vi "encoder_debug_v1.vi"() -> ()   [LabVIEW 2014]
uses:
  <vilib>/LabVIEW Targets/FPGA/cRIO/shared/nicrio_ModuleControls/nicrio_cRIO-9237_DataRatesRing.ctl
  <vilib>/LabVIEW Targets/FPGA/cRIO/shared/nicrio_ModuleControls/nicrio_cRIO-9237_ExcitationVoltageRing.ctl
  <vilib>/rvi/FXPMathLib/FxpSinAndCos/subVIs/nifxpmath_SinAndCos_SimConfig.ctl
  <vilib>/rvi/Emulation/niFpgaGetClockAttributes.vi
  <vilib>/rvi/Emulation/niFpgaSctlEmulationGetInTimedLoop.vi
  <vilib>/rvi/Emulation/niFpgaEmulationReportErrorSimple.vi
  <vilib>/rvi/Emulation/niFpgaProcessEmulError.vi
  <vilib>/rvi/interface/RandomDataEmulation/nirviRandomDataMultiElementFPGAFIFO.vi
  <instcachedir>/0/nirviRandomDataMultiElementFPGAFIFO_AD0CFC12EF974623A9C2E4184BC062B2.lvgen/nirviRandomDataMultiElementFPGAFIFO_AD0CFC12EF974623A9C2E4184BC062B2_025.vi
  <vilib>/rvi/interface/RandomDataEmulation/niFpgaRandomDataHandleErrors.vi
  <vilib>/rvi/Emulation/niFpgaCriticalErrorInLSC.vi
  <vilib>/rvi/FXPMathLib/FxpSinAndCos/simVIs/DllFxpSinAndCosTemp_sub.vi
  <vilib>/rvi/eio/common/nirviEmuTemplateMethod_errors.vi
  <vilib>/rvi/eio/common/nirviEmuTemplatePropertySet_errors.vi
  <vilib>/rvi/DataTransferAndStorage/Container/XNode/niFpgaContainer.xnode
  <vilib>/rvi/interface/RandomDataEmulation/nirviRandomDataFpgaMultiElementTemplate.vi
  <vilib>/rvi/FXPMathLib/FxpSinAndCos/XNode/nifxpmath_SinAndCos.xnode
  <vilib>/rvi/Analysis/measure/butterworth/XNode/niFpgaButterworthFilter.xnode
  <vilib>/eio/EIONode/EIONode.xnode
  <vilib>/eio/EIOPropertyNode/EIOPropertyNode.xnode
  <vilib>/rvi/eio/common/nirviEmuTemplatePropertyGet_errors.vi
  <vilib>/rvi/eio/common/nirviEmuTemplatePropertyGet_noerrors.vi
  <vilib>/rvi/eio/common/nirviEmuTemplatePropertySet_noerrors.vi
panel:
  out "omega_p2 (rad/s)":fxp<+/-,36,13>
  out "Dp2_d (mm/s)":fxp<+/-,36,13>
  out "omega_p2 (Mavg)":fxp<+/-,36,14>
  out "Dp2_d (Mavg)":fxp<+/-,36,14>
  in  "mt0_p2":u32
  out "Dp2_d (Mavg w. f.)":fxp<+/-,36,14>
  out "Dp1_d (Mavg w. f.)":fxp<+/-,36,14>
  in  "Dp_d (Mavg) coeff.":i32[](array[numeric])=[946630756, 63555534]
  in  "Dy_d (Mavg) coeff.":i32[](array[numeric])=[946630756, 63555534]
  out "omega_p2 (Mavg w. f.)":fxp<+/-,36,14>
  in  "omega_y(Mavg) coeff.":i32[](array[numeric])=[946630756, 63555534]
  out "omega_p1 (Mavg w. f)":fxp<+/-,36,14>
  in  "omega_P(Mavg) coeff.":i32[](array[numeric])=[946630756, 63555534]
  in  "FIFO":i16(ring) items=["Pitch_F+P", "imp ctrl", "Yaw_F+P"]
  out "PID (kHz)":fxp<+/-,20,10>
  in  "Set 6":bool
  in  "Set 5":bool
  in  "Set 4":bool
  in  "Set 3":bool
  in  "Set 2":bool
  in  "Set 1":bool
  out "Dp1_d (T)":fxp<+/-,36,13>
  out "omega_p1 (T)":fxp<+/-,36,13>
  out "Dp2_d (T)":fxp<+/-,36,13>
  out "omega_p2 (T)":fxp<+/-,36,13>
  out "mt_omega_p2":u32
  out "Encoder Position_p2":i32
  out "D_p2":fxp<+/-,32,7>
  out "rad_p2":fxp<+/-,33,20>
  out "D_p1":fxp<+/-,32,7>
  out "rad_p1":fxp<+/-,33,20>
  out "Encoder Position_p1":i32
  out "Dp1_d (Mavg)":fxp<+/-,36,14>
  out "omega_p1 (Mavg)":fxp<+/-,36,14>
  in  "Dp_d_M_avg_Tc (uSec)":i32
  in  "Vp. Est.":i16(ring) items=["T", "Mavg", "Mavg w. f."]
  in  "Mag. factor_p":fxp<+/-,20,3>
  in  "Belt_out_p":fxp<+/-,7,7>
  in  "Belt_in_p":fxp<+/-,6,6>
  out "Fp_dc":fxp<+/-,32,10>
  in  "Zero_p":bool
  in  "mt0_p1":u32
  in  "Dp_dd coeff.":i32[](array[numeric])=[946630756, 63555534]
  out "Dp_dd":fxp<+/-,36,25>
  out "dFp_PID":fxp<+/-,36,18>
  in  "dFp_PID coeff.":i32[](array[numeric])=[946630756, 63555534]
  out "fpt_i":fxp<+/-,34,18>
  out "Dpr_sin":fxp<+/-,22,7>
  in  "Sin offset_p":fxp<+/-,22,7>
  in  "Sin magnitude_p":fxp<+/-,21,6>
  out "Dpr_sin_dd":fxp<+/-,35,20>
  out "Dpr_sin_d":fxp<+/-,33,15>
  out "Sin omega_p":fxp<+/-,34,9>
  in  "Sin wave freq._p (Hz)":fxp<+/-,32,6>
  in  "Dpr_step":fxp<+/-,22,7>
  out "Dpr_for":fxp<+/-,22,7>
  in  "Command_p":i16(ring) items=["Step", "Sine"]
  in  "Ki_p":fxp<+/-,30,9>
  out "Fp_PID":fxp<+/-,36,16>
  in  "fp_tolorance":fxp<+,22,6>
  out "fp_tilde":fxp<+/-,33,10>
  in  "Kp_p":fxp<+/-,32,13>
  out "Fr_p":fxp<+/-,32,10>
  in  "S/F coeff_p":fxp<+/-,25,-10>
  out "va_p1":fxp<+/-,36,7>
  out "vb_p1":fxp<+/-,37,8>
  out "vq_p2_F":fxp<+/-,20,5> format="%.57g"
  out "vd_p2_F":fxp<+/-,20,5>
  in  "Stop motor_p":bool
  out "Force_p":fxp<+/-,32,10>
  in  "Strain selection_p":i16(ring) items=["Raw", "Avg.8", "Avg.8 w. filter"]
  out "Strain_p (Avg8 w. f)":fxp<+/-,36,8>
  in  "Strain_p Avg.8 coeff.":i32[](array[numeric])=[946630756, 63555534]
  out "Strain_p (Avg8)":fxp<+/-,36,4>
  out "Raw Strain_p":fxp<+/-,36,4>
  out "Mod6/AI3":fxp<+/-,36,4>
  in  "Strain gage reset_p":bool
  out "Dp1_d (mm/s)":fxp<+/-,36,13>
  out "omega_p1 (rad/s)":fxp<+/-,36,13>
  out "mt_omega_p1":u32
  in  "Encoder reset_p":bool
  out "Strain_y (Avg8 w. f)":fxp<+/-,36,8>
  in  "Strain_y Avg8 coeff.":i32[](array[numeric])=[-898916953, 1957103773, 3888751]
  out "Strain_y (Avg8)":fxp<+/-,36,4>
  out "vb_p2":fxp<+/-,38,8>
  out "va_p2":fxp<+/-,38,8>
  out "Time now(s)":fxp<+,52,14>
  out "vq_p1_F":fxp<+/-,20,5> format="%.57g"
  out "vd_p1_F":fxp<+/-,20,5>
  in  "Stop motor_y":bool
  in  "Ini coe.":bool
  out "Loop rate (kHz)":fxp<+/-,36,7>
  out "Raw Strain_y":fxp<+/-,36,4>
  in  "Strain gage reset_y":bool
  in  "Stop (Strain)":bool
  out "Mod6/AI2":fxp<+/-,36,4>
  in  "Excitation Voltage":T1 items=["2.5 Volts", "3.3 Volts", "5.0 Volts", "10.0 Volts", "External Excitation"]
  in  "Data Rate":T2=1 items=["50.000 kS/s (NI 9237)"=1, "25.000 kS/s (NI 9237)"=2, "16.667 kS/s (NI 9237)"=3, "12.500 kS/s (NI 9237)"=4, "10.000 kS/s (NI 9237)"=5, "8.333 kS/s (NI 9237)"=6, "7.143 kS/s (NI 9237)"=7, "6.250 kS/s (NI 9237)"=8, "5.556 kS/s (NI 9237)"=9, "5.000 kS/s (NI 9237)"=10, "4.545 kS/s (NI 9237)"=11, "4.167 kS/s (NI 9237)"=12, "3.846 kS/s (NI 9237)"=13, "3.571 kS/s (NI 9237)"=14, "3.333 kS/s (NI 9237)"=15, "3.125 kS/s (NI 9237)"=16, "2.941 kS/s (NI 9237)"=17, "2.778 kS/s (NI 9237)"=18, "2.632 kS/s (NI 9237)"=19, "2.500 kS/s (NI 9237)"=20, "2.381 kS/s (NI 9237)"=21, "2.273 kS/s (NI 9237)"=22, "2.174 kS/s (NI 9237)"=23, "2.083 kS/s (NI 9237)"=24, "2.000 kS/s (NI 9237)"=25, "1.923 kS/s (NI 9237)"=26, "1.852 kS/s (NI 9237)"=27, "1.786 kS/s (NI 9237)"=28, "1.724 kS/s (NI 9237)"=29, "1.667 kS/s (NI 9237)"=30, "1.613 kS/s (NI 9237)"=31]
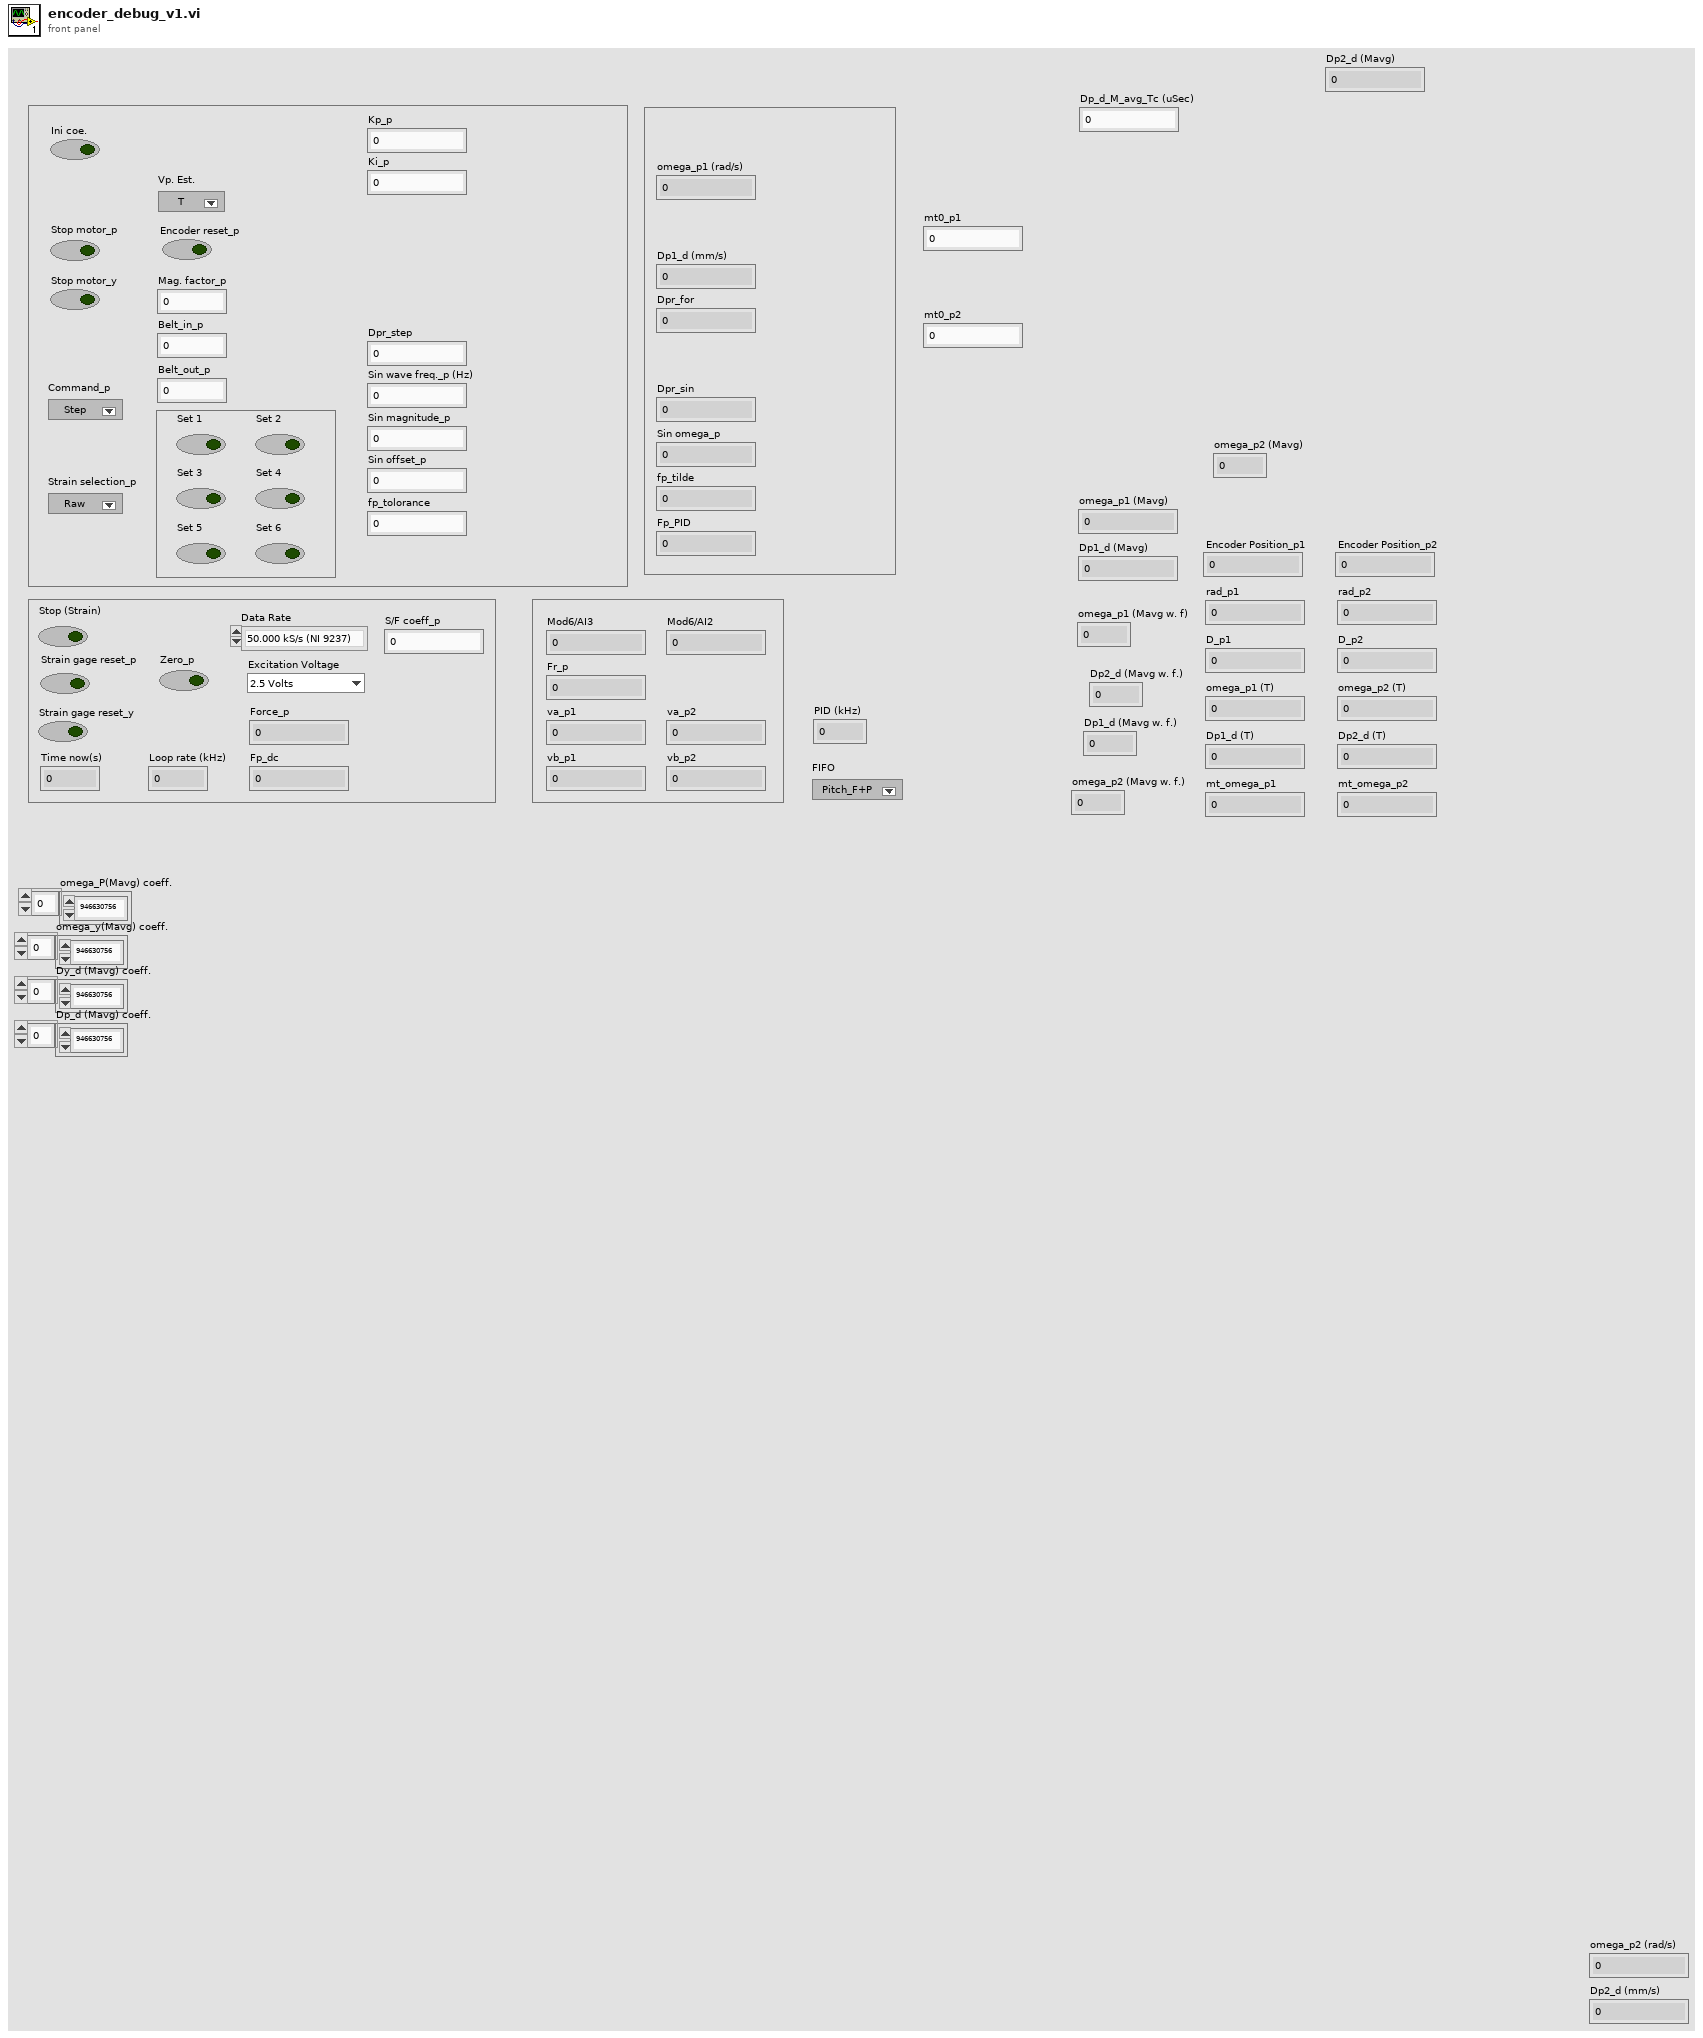
[diagram p1: front panel]
types:
  T1 = typedef "nicrio_cRIO-9237_ExcitationVoltageRing.ctl" = u8
  T2 = typedef "nicrio_cRIO-9237_DataRatesRing.ctl" = u8
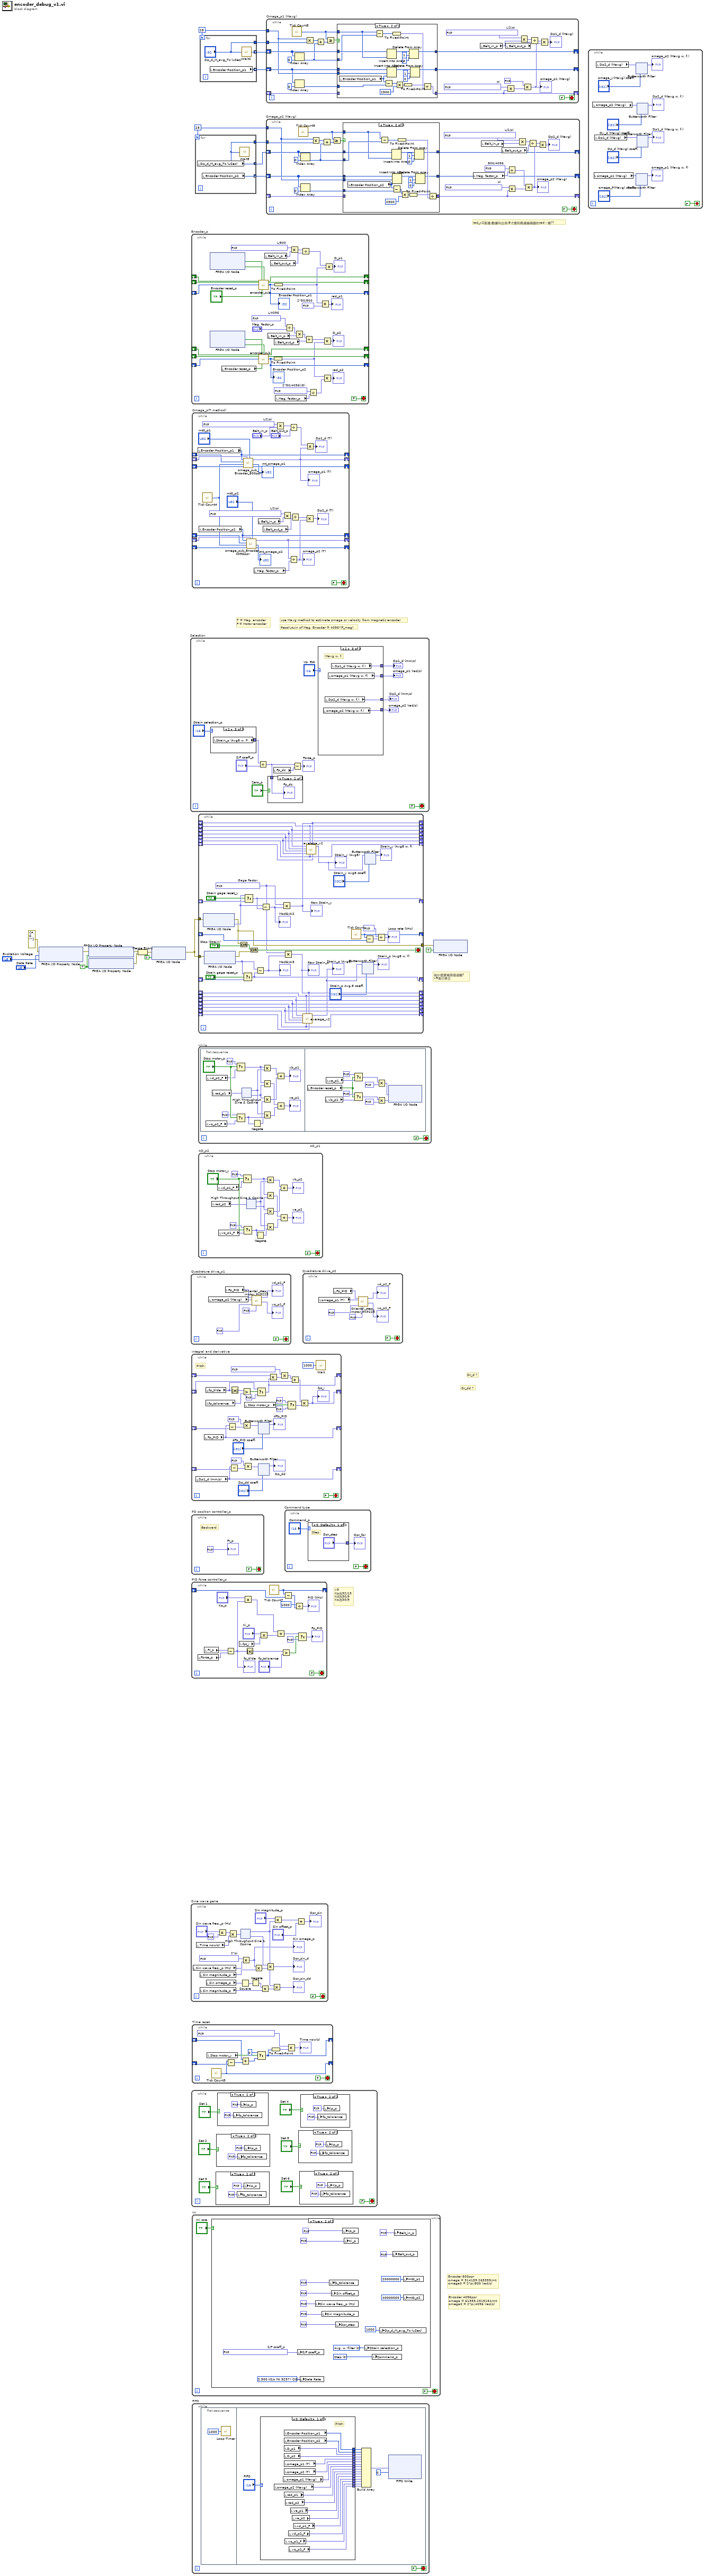
[diagram p0: block diagram]
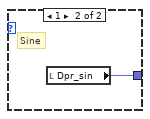
[diagram p10: hidden frame]
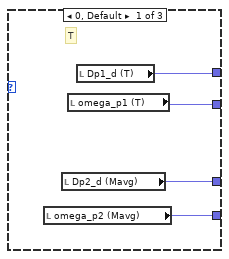
[diagram p11: hidden frame]
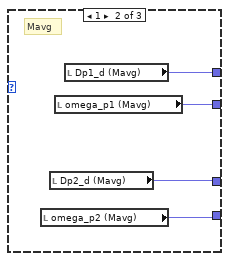
[diagram p12: hidden frame]
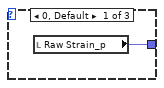
[diagram p14: hidden frame]
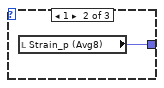
[diagram p15: hidden frame]
diagram:
  w2 = 25
  w8 = 25
  w13 = TRUE ("Half-Bridge Enable")
  # "T = Mag. encoder\nF = Motor encoder"
  # "rad_x2那邊:數據叫出來/8才會和馬達編碼器的rad一樣??"
  # "Encoder 4096ppr\nomega = 61359.2315154/mt\nomega0 = 2*pi/4096 (rad/s)"
  # "Encoder 800ppr\nomega = 314159.265359/mt\nomega0 = 2*pi/800 (rad/s)"
  # "v9\nKp改32/13\nKd改30/9\nKo改30/9"
  # "Resolutuin of Mag. Encoder = 4096*(F_mag)"
  # "use Mavg method to estimate omega or velocity from magnetic encoder"
  # "為什麼要寫兩個迴圈?\nv9後已修正"
  # "Dr_dd ?"
  # "Dr_d ?"
  n1 = xnode "FPGA I/O Property Node"("error in"=errorcluster {"status"=FALSE, "code"=0, "source"=""}, "Data Rate"="Data Rate", "Excitation Voltage"="Excitation Voltage") -> ("error out"=w18:errorcluster)  [unwired: 1 in, 1 out]
  n2 = xnode "FPGA I/O Property Node"("error in"=w18, "Half-Bridge Enable"=w13) -> ("error out"=w11:errorcluster)  [unwired: 1 in, 1 out]
  n3 = xnode "FPGA I/O Property Node"("Half-Bridge Enable"=w13) -> ("error out"=w10:errorcluster)  [unwired: 2 in, 1 out]
  n4 = Merge Errors(w11, w10) -> (w12:errorcluster)
  n5 = xnode "FPGA I/O Node"("error in"=w12, "Mod6/Start"=TRUE) -> ("error out"=w16:errorcluster)  [unwired: 1 in, 1 out]
  n6 = while "Selection" {
    stop <- FALSE stop-if-true
    n7 = case shown="2" "Strain selection_p" {
      tunnel: [w47 w48 w49] -> w32
      frame 0, Default {
        n8 = local read "Raw Strain_p"() -> (w47:fxp<+/-,36,4>)
      }
      frame 1 {
        n9 = local read "Strain_p (Avg8)"() -> (w48:fxp<+/-,36,4>)
      }
      frame 2 {
        n10 = local read "Strain_p (Avg8 w. f)"() -> (w49:fxp<+/-,36,8>)
      }
    }
    n11 = Divide(x=w32, y="S/F coeff_p") -> (x/y=w29:fxp<+/-,32,10>)
    n12 = case shown="True" "Zero_p" {
      tunnel: w29 -> [_ w46]
      frame False {
      }
      frame True {
        "Fp_dc" <- w46
      }
    }
    n13 = local read "Fp_dc"() -> (w27:fxp<+/-,32,10>)
    n14 = Subtract(x=w29, y=w27) -> (x-y=→"Force_p":fxp<+/-,33,11>)
    n15 = case shown="2" "Vp. Est." {
      tunnel: [w37 w40 w45] -> w25
      tunnel: [w36 w41 w44] -> w26
      tunnel: [w35 w38 w42] -> w22
      tunnel: [w34 w39 w43] -> w21
      frame 0, Default {
        # "T"
        n16 = local read "omega_p2 (Mavg)"() -> (w35:fxp<+/-,36,14>)
        n17 = local read "Dp2_d (Mavg)"() -> (w34:fxp<+/-,36,14>)
        n18 = local read "omega_p1 (T)"() -> (w37:fxp<+/-,36,13>)
        n19 = local read "Dp1_d (T)"() -> (w36:fxp<+/-,36,13>)
      }
      frame 1 {
        # "Mavg"
        n20 = local read "omega_p2 (Mavg)"() -> (w38:fxp<+/-,36,14>)
        n21 = local read "Dp2_d (Mavg)"() -> (w39:fxp<+/-,36,14>)
        n22 = local read "omega_p1 (Mavg)"() -> (w40:fxp<+/-,36,14>)
        n23 = local read "Dp1_d (Mavg)"() -> (w41:fxp<+/-,36,14>)
      }
      frame 2 {
        # "Mavg w. f."
        n24 = local read "omega_p2 (Mavg w. f.)"() -> (w42:fxp<+/-,36,14>)
        n25 = local read "Dp2_d (Mavg w. f.)"() -> (w43:fxp<+/-,36,14>)
        n26 = local read "omega_p1 (Mavg w. f)"() -> (w45:fxp<+/-,36,14>)
        n27 = local read "Dp1_d (Mavg w. f.)"() -> (w44:fxp<+/-,36,14>)
      }
    }
    "Dp1_d (mm/s)" <- w26
    "omega_p1 (rad/s)" <- w25
    "Dp2_d (mm/s)" <- w21
    "omega_p2 (rad/s)" <- w22
  }
  n28 = while "Quadrature drive_p1" {
    stop <- FALSE stop-if-true
    n29 = local read "omega_p2 (Mavg)"() -> (w56:fxp<+/-,36,14>)
    n30 = local read "Fp_PID"() -> (w52:fxp<+/-,36,16>)
    n31 = call "Oriental_step_motor_PKP225.vi"("F_Threshold"=fxp<+,12,12> 10.0, "dFmr"=fxp<+,1,1> 0.0 ("f"), "omega"=w56, "Fmr"=w52) -> ("vq_F"=→"vq_p1_F":fxp<+/-,20,5>, "vd_F"=→"vd_p1_F":fxp<+/-,20,5>)  [unwired: 6 in]
  }
  n32 = while "Sine wave gene" {
    stop <- FALSE stop-if-true
    w62 = fxp<+,20,3> 6.2831878662109375  # 2*pi
    n33 = local read "Sin wave freq._p (Hz)"() -> (w58:fxp<+/-,32,6>)
    n34 = local read "Time now(s)"() -> (w76:fxp<+,52,14>)
    n35 = local read "Sin magnitude_p"() -> (w59:fxp<+/-,21,6>)
    n36 = local read "Sin magnitude_p"() -> (w61:fxp<+/-,21,6>)
    n37 = local read "Sin omega_p"() -> (w60:fxp<+/-,34,9>)
    n38 = Multiply(x="Sin wave freq._p (Hz)", y=fxp<+/-,10,3> 2.0) -> (x*y=w80:fxp<+/-,42,9>)
    n39 = Multiply(x=w80, y=w76) -> (x*y=w77:fxp<+/-,41,19>)
    n40 = Square(x=w60) -> (x^2=w72:fxp<+,34,18>)
    n41 = xnode "High Throughput Sine & Cosine"("x (pi)"=w77) -> ("sin(x)"=w63:fxp<+/-,16,2>, "cos(x)"=w68:fxp<+/-,16,2>)
    n42 = Multiply(x=w62, y=w58) -> (x*y=w75:fxp<+/-,34,9>)
    "Sin omega_p" <- w75
    n43 = Negate(x=w72) -> (-x=w71:fxp<+/-,35,19>)
    n44 = Multiply(x=w75, y=w59) -> (x*y=w74:fxp<+/-,33,15>)
    n45 = Multiply(x=w71, y=w61) -> (x*y=w70:fxp<+/-,35,19>)
    n46 = Multiply(x=w68, y=w74) -> (x*y=→"Dpr_sin_d":fxp<+/-,33,15>)
    n47 = Multiply(x=w63, y=w70) -> (x*y=→"Dpr_sin_dd":fxp<+/-,35,20>)
    n48 = Multiply(x="Sin magnitude_p", y=w63) -> (x*y=w66:fxp<+/-,37,8>)
    n49 = Add(x=w66, y="Sin offset_p") -> (x+y=→"Dpr_sin":fxp<+/-,37,8>)
  }
  n50 = while "Encoder_p" {
    shift-right: [w148] -> _
    shift-left: _ -> [w147]
    shift-right: [w149] -> _
    shift-left: _ -> [w146]
    shift-right: [w143] -> _
    shift-left: _ -> [w145]
    shift-right: [w134] -> _
    shift-left: _ -> [w133]
    shift-right: [w135] -> _
    shift-left: _ -> [w136]
    shift-right: [w130] -> _
    shift-left: _ -> [w131]
    stop <- FALSE stop-if-true
    w126 = fxp<+/-,20,-5> 0.00048828125  # L/4096
    w124 = fxp<+/-,16,1> 0.0030517578125  # 2*50/4096(/8)
    w142 = fxp<+/-,20,-5> 0.002499997615814209  # L/800
    w116 = fxp<+/-,16,1> 0.125  # 2*50/800
    n51 = xnode "FPGA I/O Node"() -> ("Mod7/DIO0"=w151:bool, "Mod7/DIO1"=w150:bool)  [unwired: 2 in, 2 out]
    n52 = xnode "FPGA I/O Node"() -> ("Mod7/DIO4"=w138:bool, "Mod7/DIO5"=w137:bool)  [unwired: 2 in, 2 out]
    n53 = local read "Encoder reset_p"() -> (w132:bool)
    n54 = call "encoder_sub.vi"("A_pre"=w147, "B_pre"=w146, "Encoder Position_pre"=w145, "A input"=w151, "Encoder Position Reset"="Encoder reset_p", "B input"=w150) -> ("A"=w148:bool, "B"=w149:bool, "Encoder Position (Counts)"=w143:i32)  [unwired: 19 in]
    "Encoder Position_p1" <- w143
    n55 = call "encoder_sub.vi"("A_pre"=w133, "B_pre"=w136, "Encoder Position_pre"=w131, "A input"=w138, "Encoder Position Reset"=w132, "B input"=w137) -> ("A"=w134:bool, "B"=w135:bool, "Encoder Position (Counts)"=w130:i32)  [unwired: 19 in]
    "Encoder Position_p2" <- w130
    n56 = local read "Belt_in_p"() -> (w141:fxp<+/-,6,6>)
    n57 = local read "Belt_in_p"() -> (w127:fxp<+/-,6,6>)
    n58 = local read "Belt_out_p"() -> (w139:fxp<+/-,7,7>)
    n59 = To Fixed-Point(number=w130) -> (fixed-point=w112:fxp<+/-,32,32>)  [unwired: 1 in]
    n60 = To Fixed-Point(number=w143) -> (fixed-point=w117:fxp<+/-,32,32>)  [unwired: 1 in]
    n61 = local read "Belt_out_p"() -> (w129:fxp<+/-,7,7>)
    n62 = local read "Mag. factor_p"() -> (w123:fxp<+/-,20,3>)
    n63 = Divide(x=w126, y="Mag. factor_p") -> (x/y=w125:fxp<+/-,41,13>)
    n64 = Multiply(x=w142, y=w141) -> (x*y=w140:fxp<+/-,26,1>)
    n65 = Multiply(x=w125, y=w127) -> (x*y=w128:fxp<+/-,46,18>)
    n66 = Divide(x=w140, y=w139) -> (x/y=w119:fxp<+/-,33,1>)
    n67 = Divide(x=w128, y=w129) -> (x/y=w114:fxp<+/-,53,18>)
    n68 = Divide(x=w124, y=w123) -> (x/y=w111:fxp<+/-,32,1>)
    n69 = Multiply(x=w117, y=w116) -> (x*y=→"rad_p1":fxp<+/-,33,20>)
    n70 = Multiply(x=w114, y=w112) -> (x*y=→"D_p2":fxp<+/-,37,7>)
    n71 = Multiply(x=w112, y=w111) -> (x*y=→"rad_p2":fxp<+/-,33,20>)
    n72 = Multiply(x=w119, y=w117) -> (x*y=→"D_p1":fxp<+/-,32,7>)
  }
  n73 = while "Integral and derivative" {
    shift-right: [w175] -> _
    shift-left: _ -> [w178]
    shift-right: [w168] -> _
    shift-left: _ -> [w167]
    shift-right: [w162] -> _
    shift-left: _ -> [w161]
    shift-right: [w157] -> _
    shift-left: _ -> [w158]
    stop <- FALSE stop-if-true
    # "Pitch"
    n74 = local read "Dp1_d (mm/s)"() -> (w157:fxp<+/-,36,13>)
    n75 = local read "Fp_PID"() -> (w162:fxp<+/-,36,16>)
    n76 = local read "fp_tilde"() -> (w179:fxp<+/-,33,10>)
    n77 = local read "fp_tolorance"() -> (w182:fxp<+,22,6>)
    n78 = Subtract(x=w162, y=w161) -> (x-y=w166:fxp<+/-,37,17>)
    n79 = Subtract(x=w157, y=w158) -> (x-y=w159:fxp<+/-,37,14>)
    n80 = Absolute Value(x=w179) -> (abs(x)=w183:fxp<+,33,10>)
    n81 = Greater?(x=w183, y=w182) -> (0:w181:bool)
    n82 = Multiply(x=fxp<+,7,10> 1000.0, y=w166) -> (x*y=w164:fxp<+/-,32,18>)
    n83 = Multiply(x=fxp<+,7,10> 1000.0, y=w159) -> (x*y=w155:fxp<+/-,36,21>)
    n84 = local read "Stop motor_p"() -> (w170:bool)
    n85 = Select(t=w179, s=w181, f=fxp<+,1,1> 0.0) -> (s? t:f=w175:fxp<+/-,33,10>)
    n86 = xnode "Butterworth Filter"("input data"=w164, "scaled coefficients"="dFp_PID coeff.") -> ("output data"=→"dFp_PID":fxp<+/-,36,22>)  [unwired: 1 in]
    n87 = xnode "Butterworth Filter"("input data"=w155, "scaled coefficients"="Dp_dd coeff.") -> ("output data"=→"Dp_dd":fxp<+/-,36,25>)  [unwired: 1 in]
    n88 = Multiply(x=w178, y=w175) -> (x*y=w177:fxp<+/-,34,12>)
    n89 = Multiply(x=fxp<+/-,30,12> 0.000499725341796875, y=w177) -> (x*y=w174:fxp<+/-,34,10>)
    n90 = Select(t=fxp<+,1,1> 0.0, s=w170, f=fxp<+,1,1> 1.0) -> (s? t:f=w172:fxp<+,1,1>)
    n91 = Add(x=w174, y=w167) -> (x+y=w173:fxp<+/-,36,16>)
    n92 = Multiply(x=w173, y=w172) -> (x*y=w168:fxp<+/-,34,18>)
    "fpt_i" <- w168
    n93 = call "Wait"("Count(uSec)"=u32 1000) -> ()  [unwired: 1 out]
  }
  n94 = while "PD position controller_p" {
    stop <- FALSE stop-if-true
    # "Backward"
    "Fr_p" <- fxp<+/-,62,19> 0.0
  }
  n95 = while "PID force controller_p" {
    shift-right: [w208] -> _
    shift-left: _ -> [w207]
    stop <- FALSE stop-if-true
    n96 = local read "Force_p"() -> (w215:fxp<+/-,32,10>)
    n97 = local read "Fr_p"() -> (w216:fxp<+/-,32,10>)
    n98 = Subtract(x=w216, y=w215) -> (x-y=w213:fxp<+/-,33,11>)
    "fp_tilde" <- w213
    n99 = local read "fpt_i"() -> (w211:fxp<+/-,34,18>)
    n100 = Multiply(x="Kp_p", y=w213) -> (x*y=w203:fxp<+/-,64,23>)
    n101 = Absolute Value(x=w213) -> (abs(x)=w222:fxp<+,32,10>)
    n102 = Multiply(x="Ki_p", y=w211) -> (x*y=w210:fxp<+/-,64,27>)
    n103 = call "Tick Count7"() -> ("Tick Count(uSec)"=w208:u32)
    n104 = Add(x=w203, y=w210) -> (x+y=w209:fxp<+/-,64,27>)
    n105 = Greater?(x=w222, y="fp_tolorance") -> (0:w219:bool)
    n106 = Subtract(x=w208, y=w207) -> (x-y=w206:u32)
    n107 = Divide(x=u32 1000, y=w206) -> (x/y=→"PID (kHz)":fxp<+/-,20,7>)
    n108 = Select(t=w209, s=w219, f=fxp<+,1,1> 0.0) -> (s? t:f=→"Fp_PID":fxp<+/-,64,27>)
  }
  n109 = while {
    stop <- FALSE stop-if-true
    n110 = case shown="True" "Set 3" {
      frame False {
      }
      frame True {
        n111 = local write "fp_tolorance"(fxp<+,22,6> 3.0 ("fp_tolorance")) -> ()
        n112 = local write "Kp_p"(fxp<+/-,36,9> 100.0 ("Kp_p")) -> ()
      }
    }
    n113 = case shown="True" "Set 2" {
      frame False {
      }
      frame True {
        n114 = local write "fp_tolorance"(fxp<+,22,6> 1.5 ("fp_tolorance")) -> ()
        n115 = local write "Kp_p"(fxp<+/-,36,9> 50.0 ("Kp_p")) -> ()
      }
    }
    n116 = case shown="True" "Set 1" {
      frame False {
      }
      frame True {
        n117 = local write "fp_tolorance"(fxp<+,22,6> 3.0 ("fp_tolorance")) -> ()
        n118 = local write "Kp_p"(fxp<+/-,36,9> 50.0 ("Kp_p")) -> ()
      }
    }
    n119 = case shown="True" "Set 5" {
      frame False {
      }
      frame True {
        n120 = local write "fp_tolorance"(fxp<+,22,6> 3.0 ("fp_tolorance")) -> ()
        n121 = local write "Kp_p"(fxp<+/-,36,9> 150.0 ("Kp_p")) -> ()
      }
    }
    n122 = case shown="True" "Set 6" {
      frame False {
      }
      frame True {
        n123 = local write "fp_tolorance"(fxp<+,22,6> 1.5 ("fp_tolorance")) -> ()
        n124 = local write "Kp_p"(fxp<+/-,36,9> 150.0 ("Kp_p")) -> ()
      }
    }
    n125 = case shown="True" "Set 4" {
      frame False {
      }
      frame True {
        n126 = local write "fp_tolorance"(fxp<+,22,6> 1.5 ("fp_tolorance")) -> ()
        n127 = local write "Kp_p"(fxp<+/-,36,9> 100.0 ("Kp_p")) -> ()
      }
    }
  }
  n128 = while "Omega_p(T method)" {
    shift-right: [w273] -> _
    shift-left: _ -> [w271]
    shift-right: [w254] -> _
    shift-left: _ -> [w272]
    shift-right: [w269] -> _
    shift-left: _ -> [w270]
    shift-right: [w247] -> _
    shift-left: _ -> [w246]
    shift-right: [w242] -> _
    shift-left: _ -> [w244]
    shift-right: [w250] -> _
    shift-left: _ -> [w249]
    stop <- FALSE stop-if-true
    w261 = fxp<+/-,32,0> 0.3183098859153688  # L/2/pi
    w266 = fxp<+/-,32,0> 0.3183098859153688  # L/2/pi
    n129 = local read "Encoder Position_p1"() -> (w273:i32)
    n130 = local read "Encoder Position_p2"() -> (w247:i32)
    n131 = call "Tick Count4"() -> ("Tick Count(Ticks)"=w248:u32)
    n132 = call "omega_sub_Encoder_800ppr.vi"("mt0"="mt0_p1", "omega_pre"=w272, "ticks_m_pre"=w270, "ticks"=w248, "count_pre"=w271, "count"=w273) -> ("ticks_m"=w269:u32, "mt"=→"mt_omega_p1":u32, "omega"=w254:fxp<+/-,36,13>)  [unwired: 3 in]
    "omega_p1 (T)" <- w254
    n133 = call "omega_sub_Encoder_4096ppr.vi"("mt0"="mt0_p2", "omega_pre"=w244, "ticks_m_pre"=w249, "ticks"=w248, "count_pre"=w246, "count"=w247) -> ("ticks_m"=w250:u32, "mt"=→"mt_omega_p2":u32, "omega"=w242:fxp<+/-,36,13>)  [unwired: 3 in]
    n134 = local read "Mag. factor_p"() -> (w262:fxp<+/-,20,3>)
    n135 = local read "Belt_in_p"() -> (w259:fxp<+/-,6,6>)
    n136 = local read "Belt_out_p"() -> (w258:fxp<+/-,7,7>)
    n137 = Multiply(x=w266, y="Belt_in_p") -> (x*y=w264:fxp<+/-,38,6>)
    n138 = Multiply(x=w261, y=w259) -> (x*y=w260:fxp<+/-,38,6>)
    n139 = Divide(x=w264, y="Belt_out_p") -> (x/y=w255:fxp<+/-,20,1>)
    n140 = Divide(x=w242, y=w262) -> (x/y=w243:fxp<+/-,57,31>)
    "omega_p2 (T)" <- w243
    n141 = Divide(x=w260, y=w258) -> (x/y=w253:fxp<+/-,45,6>)
    n142 = Multiply(x=w253, y=w243) -> (x*y=→"Dp2_d (T)":fxp<+/-,36,13>)
    n143 = Multiply(x=w255, y=w254) -> (x*y=→"Dp1_d (T)":fxp<+/-,36,13>)
  }
  n144 = while "Time reset" {
    shift-right: [w283] -> _
    shift-left: _ -> [w284]
    shift-right: [w278] -> _
    shift-left: _ -> [w279]
    stop <- FALSE stop-if-true
    n145 = local read "Stop motor_y"() -> (w285:bool)
    n146 = call "Tick Count3"() -> ("Tick Count(uSec)"=w283:u32)
    n147 = Subtract(x=w283, y=w284) -> (x-y=w282:u32)
    n148 = Add(x=w279, y=w282) -> (x+y=w281:u32)
    n149 = Select(t=u32 0, s=w285, f=w281) -> (s? t:f=w278:u32)
    n150 = To Fixed-Point(number=w278) -> (fixed-point=w277:fxp<+,32,32>)  [unwired: 1 in]
    n151 = Multiply(x=fxp<+,20,-18> 1.0000003385357559e-06, y=w277) -> (x*y=→"Time now(s)":fxp<+,52,14>)
  }
  n152 = while "Ini" {
    stop <- FALSE stop-if-true
    n153 = case shown="True" "Ini coe." {
      frame False {
      }
      frame True {
        w290 = T2 20 items=["50.000 kS/s (NI 9237)"=1, "25.000 kS/s (NI 9237)"=2, "16.667 kS/s (NI 9237)"=3, "12.500 kS/s (NI 9237)"=4, "10.000 kS/s (NI 9237)"=5, "8.333 kS/s (NI 9237)"=6, "7.143 kS/s (NI 9237)"=7, "6.250 kS/s (NI 9237)"=8, "5.556 kS/s (NI 9237)"=9, "5.000 kS/s (NI 9237)"=10, "4.545 kS/s (NI 9237)"=11, "4.167 kS/s (NI 9237)"=12, "3.846 kS/s (NI 9237)"=13, "3.571 kS/s (NI 9237)"=14, "3.333 kS/s (NI 9237)"=15, "3.125 kS/s (NI 9237)"=16, "2.941 kS/s (NI 9237)"=17, "2.778 kS/s (NI 9237)"=18, "2.632 kS/s (NI 9237)"=19, "2.500 kS/s (NI 9237)"=20, "2.381 kS/s (NI 9237)"=21, "2.273 kS/s (NI 9237)"=22, "2.174 kS/s (NI 9237)"=23, "2.083 kS/s (NI 9237)"=24, "2.000 kS/s (NI 9237)"=25, "1.923 kS/s (NI 9237)"=26, "1.852 kS/s (NI 9237)"=27, "1.786 kS/s (NI 9237)"=28, "1.724 kS/s (NI 9237)"=29, "1.667 kS/s (NI 9237)"=30, "1.613 kS/s (NI 9237)"=31] ("Data Rate")
        w301 = i16 0 items=["Step", "Sine"] ("Command_p")
        w302 = i16 2 items=["Raw", "Avg.", "Avg. w. filter"] ("Strain selection_p")
        w303 = fxp<+/-,25,-10> 5.851034075021744e-07  # S/F coeff_p
        n154 = local write "S/F coeff_p"(w303) -> ()
        n155 = local write "Data Rate"(w290) -> ()
        n156 = local write "Sin wave freq._p (Hz)"(fxp<+/-,32,6> 1.0 ("Sin wave freq._p (Hz)")) -> ()
        n157 = local write "Sin magnitude_p"(fxp<+/-,21,6> 5.0 ("Sin magnitude_p")) -> ()
        n158 = local write "fp_tolorance"(fxp<+,22,6> 5.0 ("fp_tolorance")) -> ()
        n159 = local write "Sin offset_p"(fxp<+/-,22,7> 0.0 ("Sin offset_p")) -> ()
        n160 = local write "Dpr_step"(fxp<+/-,22,7> 0.0 ("Dpr_step")) -> ()
        n161 = local write "Kp_p"(fxp<+/-,36,9> 30.0 ("Kp_p")) -> ()
        n162 = local write "Ki_p"(fxp<+/-,36,9> 0.0 ("Ki_p")) -> ()
        n163 = local write "Strain selection_p"(w302) -> ()
        n164 = local write "Command_p"(w301) -> ()
        n165 = local write "Dp_d_M_avg_Tc (uSec)"(u32 1000 ("D_d_M_avg_Tc (uSec)")) -> ()
        n166 = local write "Belt_out_p"(fxp<+/-,7,7> 36.0 ("Belt_op")) -> ()
        n167 = local write "Belt_in_p"(fxp<+/-,6,6> 14.0 ("Belt_mp")) -> ()
        n168 = local write "mt0_p1"(u32 20000000 ("mt0_p1")) -> ()
        n169 = local write "mt0_p2"(u32 40000000 ("mt0_p2")) -> ()
      }
    }
  }
  n170 = while "FIFO" {
    stop <- FALSE stop-if-true
    n171 = flat-sequence {
      frame #0 {
        n172 = call "Loop Timer"("Count(uSec)"=u32 1000) -> ()  [unwired: 1 out]
      }
      frame #1 {
        n173 = case shown="0, Default" "FIFO" {
          tunnel: [w340] -> w324
          tunnel: [w339] -> w323
          tunnel: [w338] -> w322
          tunnel: [w337] -> w321
          tunnel: [w334] -> w319
          tunnel: [w335] -> w318
          tunnel: [w336] -> w317
          tunnel: [w332] -> w316
          tunnel: [w331] -> w315
          tunnel: [w330] -> w314
          tunnel: [w329] -> w313
          tunnel: [w328] -> w312
          tunnel: [w327] -> w311
          tunnel: [w326] -> w310
          tunnel: [w325] -> w309
          tunnel: [w333] -> w307
          frame 0, Default {
            # "Pitch"
            n174 = local read "omega_p2 (Mavg)"() -> (w333:fxp<+/-,36,14>)
            n175 = local read "omega_p1 (Mavg)"() -> (w334:fxp<+/-,36,14>)
            n176 = local read "Encoder Position_p1"() -> (w340:i32)
            n177 = local read "Encoder Position_p2"() -> (w339:i32)
            n178 = local read "D_p1"() -> (w338:fxp<+/-,32,7>)
            n179 = local read "D_p2"() -> (w337:fxp<+/-,32,7>)
            n180 = local read "omega_p1 (T)"() -> (w336:fxp<+/-,36,13>)
            n181 = local read "omega_p2 (T)"() -> (w335:fxp<+/-,36,13>)
            n182 = local read "rad_p1"() -> (w332:fxp<+/-,33,20>)
            n183 = local read "vq_p1_F"() -> (w326:fxp<+/-,20,5>)
            n184 = local read "rad_p2"() -> (w331:fxp<+/-,33,20>)
            n185 = local read "vd_p2_F"() -> (w327:fxp<+/-,20,5>)
            n186 = local read "vq_p2_F"() -> (w325:fxp<+/-,20,5>)
            n187 = local read "va_p1"() -> (w330:fxp<+/-,36,7>)
            n188 = local read "va_p2"() -> (w329:fxp<+/-,38,8>)
            n189 = local read "vd_p1_F"() -> (w328:fxp<+/-,20,5>)
          }
        }
        n190 = Build Array(w324, w323, w322, w321, w317, w318, w319, w307, w316, w315, w314, w313, w312, w311, w310, w309) -> (w308:fxp<+/-,62,32>[])
        n191 = xnode ("FIFO Write")("Element"=w308, "Timeout"=0) -> ()  [unwired: 1 in, 2 out]
      }
    }
  }
  n192 = for {
    N: w2 -> [_]
    tunnel: [w342] -> w4 mode=indexing
    tunnel: [w341] -> w3 mode=indexing
    tunnel: [w341] -> w1
    n193 = local read "Dp_d_M_avg_Tc (uSec)"() -> (w341:i32)
    n194 = local read "Encoder Position_p2"() -> (w342:i32)
    n195 = call "Wait5"("Count(uSec)"=w341) -> ()  [unwired: 1 out]
  }
  n196 = while {
    tunnel: w16 -> [w387]
    tunnel: [w361] -> w9
    shift-right: [w385] -> _
    shift-left: _ -> [w386]
    shift-right: [w381] -> _
    shift-left: _ -> [w382]
    shift-right: [w376] -> _
    shift-left: _ -> [w375]
    shift-right: [w375] -> _
    shift-left: _ -> [w374]
    shift-right: [w374] -> _
    shift-left: _ -> [w373]
    shift-right: [w373] -> _
    shift-left: _ -> [w372]
    shift-right: [w372] -> _
    shift-left: _ -> [w371]
    shift-right: [w371] -> _
    shift-left: _ -> [w370]
    shift-right: [w370] -> _
    shift-left: _ -> [w369]
    tunnel: w16 -> [w365]
    shift-right: [w358] -> _
    shift-left: _ -> [w359]
    shift-right: [w354] -> _
    shift-left: _ -> [w353]
    shift-right: [w353] -> _
    shift-left: _ -> [w352]
    shift-right: [w352] -> _
    shift-left: _ -> [w351]
    shift-right: [w351] -> _
    shift-left: _ -> [w350]
    shift-right: [w350] -> _
    shift-left: _ -> [w349]
    shift-right: [w349] -> _
    shift-left: _ -> [w348]
    shift-right: [w348] -> _
    shift-left: _ -> [w347]
    stop <- w362 stop-if-true
    w356 = fxp<+,20,2> 2.115001678466797  # Gage Factor
    n197 = xnode "FPGA I/O Node"("error in"=w387) -> ("error out"=w361:errorcluster, "Mod6/AI2"=w383:fxp<+/-,24,-4>)  [unwired: 1 in, 1 out]
    n198 = xnode "FPGA I/O Node"("error in"=w365) -> ("error out"=w363:errorcluster, "Mod6/AI3"=w357:fxp<+/-,24,-4>)  [unwired: 1 in, 1 out]
    n199 = Or(x=w361, y="Stop (Strain)") -> (x .or. y?=w364:bool)
    n200 = Select(t=w357, s="Strain gage reset_p", f=w359) -> (s? t:f=w358:fxp<+/-,24,-4>)
    n201 = Select(t=w383, s="Strain gage reset_y", f=w386) -> (s? t:f=w385:fxp<+/-,24,-4>)
    n202 = Or(x=w364, y=w363) -> (x .or. y?=w362:bool)
    n203 = Subtract(x=w357, y=w358) -> (x-y=w355:fxp<+/-,30,-3>)
    "Mod6/AI3" <- w355
    n204 = Subtract(x=w383, y=w385) -> (x-y=w384:fxp<+/-,30,-3>)
    "Mod6/AI2" <- w384
    n205 = Multiply(x=w356, y=w384) -> (x*y=w376:fxp<+/-,41,6>)
    "Raw Strain_y" <- w376
    n206 = Multiply(x=w356, y=w355) -> (x*y=w354:fxp<+/-,50,-1>)
    "Raw Strain_p" <- w354
    n207 = call "average_v2.vi"("Numeric 8"=w347, "Numeric"=w354, "Numeric 7"=w348, "Numeric 2"=w353, "Numeric 6"=w349, "Numeric 5"=w350, "Numeric 4"=w351, "Numeric 3"=w352) -> ("Mean (8pt)"=w346:fxp<+/-,32,4>)  [unwired: 1 in, 2 out]
    "Strain_p (Avg8)" <- w346
    n208 = call "average_v2.vi"("Numeric 8"=w369, "Numeric"=w376, "Numeric 7"=w370, "Numeric 2"=w375, "Numeric 6"=w371, "Numeric 5"=w372, "Numeric 4"=w373, "Numeric 3"=w374) -> ("Mean (8pt)"=w368:fxp<+/-,32,4>)  [unwired: 1 in, 2 out]
    "Strain_y (Avg8)" <- w368
    n209 = call "Tick Count"() -> ("Tick Count(uSec)"=w381:u32)
    n210 = xnode "Butterworth Filter"("input data"=w346, "scaled coefficients"="Strain_p Avg.8 coeff.") -> ("output data"=→"Strain_p (Avg8 w. f)":fxp<+/-,36,8>)  [unwired: 1 in]
    n211 = xnode "Butterworth Filter"("input data"=w368, "scaled coefficients"="Strain_y Avg8 coeff.") -> ("output data"=→"Strain_y (Avg8 w. f)":fxp<+/-,32,4>)  [unwired: 1 in]
    n212 = Subtract(x=w381, y=w382) -> (x-y=w379:fxp<+/-,32,16>)
    n213 = Divide(x=fxp<+,7,10> 1000.0, y=w379) -> (x/y=→"Loop rate (kHz)":fxp<+/-,40,27>)
  }
  n214 = while "AO_p1" {
    stop <- FALSE stop-if-true
    n215 = flat-sequence {
      frame #0 {
        n216 = local read "vq_p2_F"() -> (w417:fxp<+/-,20,5>)
        n217 = local read "vd_p2_F"() -> (w419:fxp<+/-,20,5>)
        n218 = local read "rad_p1"() -> (w416:fxp<+/-,33,20>)
        n219 = Select(t=fxp<+/-,20,5> 0.0, s="Stop motor_p", f=w419) -> (s? t:f=w408:fxp<+/-,20,5>)
        n220 = Select(t=fxp<+,1,1> 0.0, s="Stop motor_p", f=w417) -> (s? t:f=w407:fxp<+/-,20,5>)
        n221 = xnode "High Throughput Sine & Cosine"("x (pi)"=w416) -> ("sin(x)"=w410:fxp<+/-,16,2>, "cos(x)"=w409:fxp<+/-,16,2>)
        n222 = Negate(x=w407) -> (-x=w415:fxp<+/-,21,6>)
        n223 = Multiply(x=w408, y=w410) -> (x*y=w414:fxp<+/-,36,7>)
        n224 = Multiply(x=w408, y=w409) -> (x*y=w412:fxp<+/-,36,7>)
        n225 = Multiply(x=w409, y=w407) -> (x*y=w413:fxp<+/-,36,7>)
        n226 = Multiply(x=w410, y=w415) -> (x*y=w411:fxp<+/-,35,6>)
        n227 = Add(x=w414, y=w413) -> (x+y=→"vb_p1":fxp<+/-,37,8>)
        n228 = Add(x=w412, y=w411) -> (x+y=→"va_p1":fxp<+/-,36,7>)
      }
      frame #1 {
        n229 = local read "Encoder reset_p"() -> (w452:bool)
        n230 = local read "vb_p1"() -> (w453:fxp<+/-,37,8>)
        n231 = local read "va_p1"() -> (w454:fxp<+/-,36,7>)
        n232 = Select(t=fxp<+,2,2> 3.0, s=w452, f=w454) -> (s? t:f=w460:fxp<+/-,36,7>)
        n233 = Select(t=fxp<+,1,1> 0.0, s=w452, f=w453) -> (s? t:f=w459:fxp<+/-,37,8>)
        n234 = Multiply(x=w460, y=fxp<+/-,1,0> -0.5) -> (x*y=w455:fxp<+/-,36,6>)
        n235 = Multiply(x=w459, y=fxp<+/-,1,0> -0.5) -> (x*y=w456:fxp<+/-,36,6>)
        n236 = xnode "FPGA I/O Node"("Mod8/AO0"=w455, "Mod8/AO1"=w456) -> ()  [unwired: 2 in, 2 out]
      }
    }
  }
  n237 = while "AO_p2" {
    stop <- FALSE stop-if-true
    n238 = local read "rad_p2"() -> (w463:fxp<+/-,33,20>)
    n239 = local read "vd_p1_F"() -> (w465:fxp<+/-,20,5>)
    n240 = local read "vq_p1_F"() -> (w466:fxp<+/-,20,5>)
    n241 = Select(t=fxp<+/-,20,5> 0.0, s="Stop motor_y", f=w465) -> (s? t:f=w471:fxp<+/-,20,5>)
    n242 = Select(t=fxp<+/-,20,5> 0.0, s="Stop motor_y", f=w466) -> (s? t:f=w472:fxp<+/-,20,5>)
    n243 = xnode "High Throughput Sine & Cosine"("x (pi)"=w463) -> ("sin(x)"=w469:fxp<+/-,17,2>, "cos(x)"=w470:fxp<+/-,17,2>)
    n244 = Negate(x=w472) -> (-x=w473:fxp<+/-,21,6>)
    n245 = Multiply(x=w471, y=w469) -> (x*y=w474:fxp<+/-,37,7>)
    n246 = Multiply(x=w471, y=w470) -> (x*y=w476:fxp<+/-,37,7>)
    n247 = Multiply(x=w470, y=w472) -> (x*y=w475:fxp<+/-,37,7>)
    n248 = Multiply(x=w469, y=w473) -> (x*y=w477:fxp<+/-,36,6>)
    n249 = Add(x=w474, y=w475) -> (x+y=→"vb_p2":fxp<+/-,38,8>)
    n250 = Add(x=w476, y=w477) -> (x+y=→"va_p2":fxp<+/-,37,7>)
  }
  n251 = for {
    N: w8 -> [_]
    tunnel: ["Dp_d_M_avg_Tc (uSec)"] -> w5
    tunnel: [w512] -> w7 mode=indexing
    tunnel: [w511] -> w6 mode=indexing
    n252 = local read "Encoder Position_p1"() -> (w511:i32)
    n253 = call "Wait2"("Count(uSec)"="Dp_d_M_avg_Tc (uSec)") -> ("Tick Count(uSec)"=w512:u32)
  }
  n254 = while "Omega_p2 (Mavg)" {
    shift-right: [w515] -> _
    shift-left: w4 -> [w536]
    shift-right: [w516] -> _
    shift-left: w3 -> [w534]
    shift-right: [w520] -> _
    shift-left: _ -> [w518]
    tunnel: w2 -> [w532]
    tunnel: w1 -> [w537]
    stop <- FALSE stop-if-true
    w521 = fxp<+/-,27,3> 3.1415926814079285  # pi
    w524 = fxp<+,32,0> 0.1953125  # 800/4096
    w529 = fxp<+/-,32,0> 0.3183098859153688  # L/2/pi
    n255 = call "Tick Count9"() -> ("Tick Count(uSec)"=w531:u32)
    n256 = Index Array(array=w534, index=0) -> (element=w533:i32)
    n257 = Index Array(array=w536, index=0) -> (element=w535:i32)
    n258 = Multiply(x=w532, y=w537) -> (x*y=w540:i32)
    n259 = Add(x=w540, y=w533) -> (x+y=w539:i32)
    n260 = Greater Or Equal?(x=w531, y=w539) -> (x >= y?=w538:bool)
    n261 = case shown="True" w538 {
      tunnel: w536 -> [w544 w559]
      tunnel: w535 -> [_ w551]
      tunnel: w534 -> [w545 w560]
      tunnel: w533 -> [_ w561]
      tunnel: w532 -> [_ w558]
      tunnel: w531 -> [_ w546]
      tunnel: [w544 w549] -> w515
      tunnel: [w545 w548] -> w516
      tunnel: [w543 w547] -> w520
      tunnel: w518 -> [w543 _]
      frame False {
      }
      frame True {
        n262 = local read "Encoder Position_p2"() -> (w550:i32)
        n263 = Subtract(x=w546, y=w561) -> (x-y=w562:u32)
        n264 = Insert Into Array(array=w560, new element=w546) -> (w564:i32[])  [unwired: 1 in]
        n265 = Subtract(x=w550, y=w551) -> (x-y=w555:i32)
        n266 = Insert Into Array(array=w559, index=w558, new element=w550) -> (w565:i32[])
        n267 = To Fixed-Point(number=w562) -> (fixed-point=w552:fxp<+,32,32>)  [unwired: 1 in]
        n268 = Multiply(x=w555, y=2500) -> (x*y=w556:i32)
        n269 = To Fixed-Point(number=w556) -> (fixed-point=w557:fxp<+/-,32,32>)  [unwired: 1 in]
        n270 = Delete From Array(array=w564, length=1, index=0) -> (array with subset deleted=w548:i32[])  [unwired: 1 out]
        n271 = Delete From Array(array=w565, length=1, index=0) -> (array with subset deleted=w549:i32[])  [unwired: 1 out]
        n272 = Divide(x=w557, y=w552) -> (x/y=w547:fxp<+/-,64,32>)
      }
    }
    n273 = local read "Mag. factor_p"() -> (w523:fxp<+/-,20,3>)
    n274 = local read "Belt_in_p"() -> (w526:fxp<+/-,6,6>)
    n275 = local read "Belt_out_p"() -> (w525:fxp<+/-,7,7>)
    n276 = Divide(x=w524, y=w523) -> (x/y=w514:fxp<+/-,32,1>)
    n277 = Multiply(x=w521, y=w520) -> (x*y=w522:fxp<+/-,64,35>)
    n278 = Multiply(x=w529, y=w526) -> (x*y=w530:fxp<+/-,38,6>)
    n279 = Multiply(x=w514, y=w522) -> (x*y=w517:fxp<+/-,64,36>)
    "omega_p2 (Mavg)" <- w517
    n280 = Divide(x=w530, y=w525) -> (x/y=w528:fxp<+/-,45,6>)
    n281 = Multiply(x=w528, y=w517) -> (x*y=→"Dp2_d (Mavg)":fxp<+/-,64,41>)
  }
  n282 = while "Omega_p1 (Mavg)" {
    tunnel: w8 -> [w586]
    shift-right: [w584] -> _
    shift-left: w7 -> [w589]
    shift-right: [w583] -> _
    shift-left: w6 -> [w585]
    shift-right: [w582] -> _
    shift-left: _ -> [w581]
    tunnel: w5 -> [w579]
    stop <- FALSE stop-if-true
    w573 = fxp<+/-,27,3> 3.1415926814079285  # pi
    w572 = fxp<+/-,32,0> 0.3183098859153688  # L/2/pi
    n283 = call "Tick Count5"() -> ("Tick Count(uSec)"=w590:u32)
    n284 = Index Array(array=w589, index=0) -> (element=w588:u32)
    n285 = Index Array(array=w585, index=0) -> (element=w587:i32)
    n286 = Multiply(x=w586, y=w579) -> (x*y=w592:i32)
    n287 = Add(x=w592, y=w588) -> (x+y=w591:u32)
    n288 = Greater Or Equal?(x=w590, y=w591) -> (x >= y?=w580:bool)
    n289 = case shown="True" w580 {
      tunnel: w590 -> [_ w613]
      tunnel: w586 -> [_ w610]
      tunnel: w589 -> [w597 w612]
      tunnel: w588 -> [_ w611]
      tunnel: w587 -> [_ w607]
      tunnel: w585 -> [w596 w609]
      tunnel: [w595 w605] -> w582
      tunnel: [w597 w604] -> w584
      tunnel: [w596 w603] -> w583
      tunnel: w581 -> [w595 _]
      frame False {
      }
      frame True {
        n290 = local read "Encoder Position_p1"() -> (w606:i32)
        n291 = Subtract(x=w613, y=w611) -> (x-y=w614:u32)
        n292 = Subtract(x=w606, y=w607) -> (x-y=w599:i32)
        n293 = Insert Into Array(array=w612, new element=w613) -> (w616:u32[])  [unwired: 1 in]
        n294 = Insert Into Array(array=w609, index=w610, new element=w606) -> (w617:i32[])
        n295 = To Fixed-Point(number=w614) -> (fixed-point=w601:fxp<+,32,32>)  [unwired: 1 in]
        n296 = Multiply(x=w599, y=2500) -> (x*y=w600:i32)
        n297 = To Fixed-Point(number=w600) -> (fixed-point=w608:fxp<+/-,32,32>)  [unwired: 1 in]
        n298 = Delete From Array(array=w616, length=1, index=0) -> (array with subset deleted=w604:u32[])  [unwired: 1 out]
        n299 = Delete From Array(array=w617, length=1, index=0) -> (array with subset deleted=w603:i32[])  [unwired: 1 out]
        n300 = Divide(x=w608, y=w601) -> (x/y=w605:fxp<+/-,64,32>)
      }
    }
    n301 = local read "Belt_in_p"() -> (w577:fxp<+/-,6,6>)
    n302 = local read "Belt_out_p"() -> (w576:fxp<+/-,7,7>)
    n303 = Multiply(x=w573, y=w582) -> (x*y=w578:fxp<+/-,64,35>)
    n304 = Multiply(x=w572, y=w577) -> (x*y=w575:fxp<+/-,38,6>)
    n305 = Multiply(x=fxp<+/-,2,2> 1.0 ("f"), y=w578) -> (x*y=w571:fxp<+/-,64,37>)
    "omega_p1 (Mavg)" <- w571
    n306 = Divide(x=w575, y=w576) -> (x/y=w570:fxp<+/-,45,6>)
    n307 = Multiply(x=w570, y=w571) -> (x*y=→"Dp1_d (Mavg)":fxp<+/-,64,42>)
  }
  n308 = while "Command type" {
    stop <- FALSE stop-if-true
    n309 = case shown="0, Default" "Command_p" {
      tunnel: ["Dpr_step" w624] -> w621
      frame 0, Default {
        # "Step"
      }
      frame 1 {
        # "Sine"
        n310 = local read "Dpr_sin"() -> (w624:fxp<+/-,22,7>)
      }
    }
    "Dpr_for" <- w621
  }
  n311 = while "Quadrature drive_p2" {
    stop <- FALSE stop-if-true
    n312 = local read "omega_p1 (T)"() -> (w631:fxp<+/-,36,13>)
    n313 = local read "Fp_PID"() -> (w627:fxp<+/-,36,16>)
    n314 = call "Oriental_step_motor_PKP225.vi"("F_Threshold"=fxp<+,12,12> 10.0, "dFmr"=fxp<+,1,1> 0.0 ("f"), "omega"=w631, "Fmr"=w627) -> ("vq_F"=→"vq_p2_F":fxp<+/-,20,5>, "vd_F"=→"vd_p2_F":fxp<+/-,20,5>)  [unwired: 6 in]
  }
  n315 = xnode "FPGA I/O Node"("error in"=w9, "Mod6/Stop"=TRUE) -> ()  [unwired: 1 in, 2 out]
  n316 = while {
    stop <- FALSE stop-if-true
    n317 = local read "omega_p2 (Mavg)"() -> (w637:fxp<+/-,36,14>)
    n318 = local read "omega_p1 (Mavg)"() -> (w644:fxp<+/-,36,14>)
    n319 = local read "Dp1_d (Mavg)"() -> (w636:fxp<+/-,36,14>)
    n320 = local read "Dp2_d (Mavg)"() -> (w640:fxp<+/-,36,14>)
    n321 = xnode "Butterworth Filter"("input data"=w640, "scaled coefficients"="omega_y(Mavg) coeff.") -> ("output data"=→"omega_p2 (Mavg w. f.)":fxp<+/-,36,18>)  [unwired: 1 in]
    n322 = xnode "Butterworth Filter"("input data"=w644, "scaled coefficients"="omega_P(Mavg) coeff.") -> ("output data"=→"omega_p1 (Mavg w. f)":fxp<+/-,36,18>)  [unwired: 1 in]
    n323 = xnode "Butterworth Filter"("input data"=w637, "scaled coefficients"="Dy_d (Mavg) coeff.") -> ("output data"=→"Dp2_d (Mavg w. f.)":fxp<+/-,36,18>)  [unwired: 1 in]
    n324 = xnode "Butterworth Filter"("input data"=w636, "scaled coefficients"="Dp_d (Mavg) coeff.") -> ("output data"=→"Dp1_d (Mavg w. f.)":fxp<+/-,36,18>)  [unwired: 1 in]
  }
